vi "Run Runnable.vi"(8 "error in (no error)":errorcluster, 10 "Runnable":refnum<class "Runnable.lvclass">, 11 "Test Runner":refnum<class "Test Runner V2.lvclass">) -> (0 "error out":errorcluster)   [LabVIEW 2020, in "Test Runner V2.lvclass"]
uses:
  Test Runner V2.lvclass
  Run/Runnable.lvclass
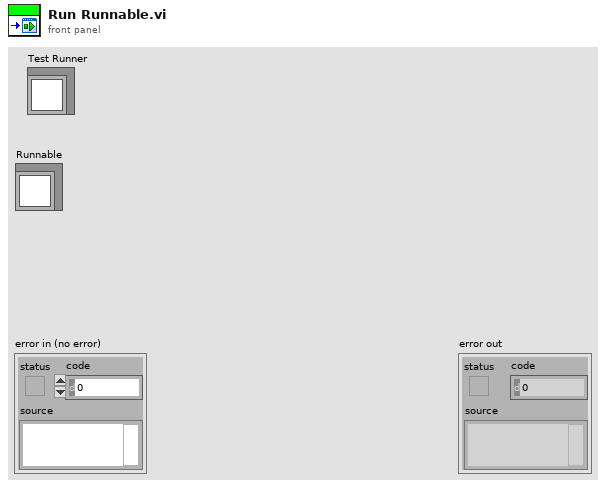
[diagram p1: front panel]
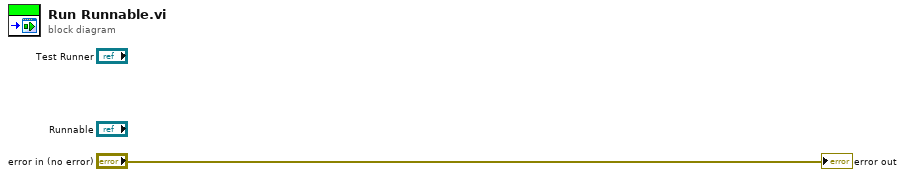
[diagram p0: block diagram]
diagram:
  "error out" <- "error in (no error)"
